vi "Open.vi"(8 "error in (no error)":errorcluster, 10 "address":string, 11 "Inst.Xeryon-Rotator in":refnum<class "Inst.Xeryon-Rotator.lvclass">) -> (0 "error out":errorcluster, 3 "Inst.Xeryon-Rotator out":refnum<class "Inst.Xeryon-Rotator.lvclass">)   [LabVIEW 2019, in "Inst.Xeryon-Rotator.lvclass"]
uses:
  Inst.Xeryon-Rotator.lvclass
  <userlib>/LevyLab/Instrument Framework/Instrument/Instrument.lvclass
  <userlib>/LevyLab/Instrument Framework/Instrument Types/Cryostat/Instrument.Cryostat.lvclass
  C:/Program Files (x86)/National Instruments/LabVIEW 2019/user.lib/LevyLab/Instrument Framework/Instrument Types/Cryostat/Instrument.Cryostat.lvclass
  C:/Program Files (x86)/National Instruments/LabVIEW 2019/user.lib/LevyLab/Instrument Framework/Instrument/Instrument.lvclass
  C:/Program Files (x86)/National Instruments/LabVIEW 2019/vi.lib/JKI/JKI SMO/SMO/SMO.lvclass
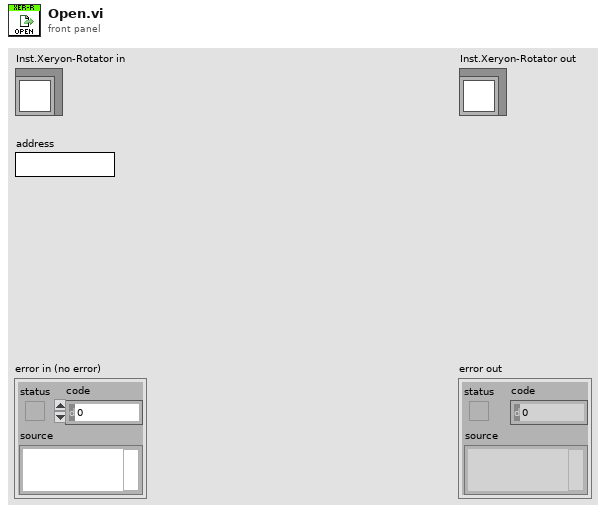
[diagram p1: front panel]
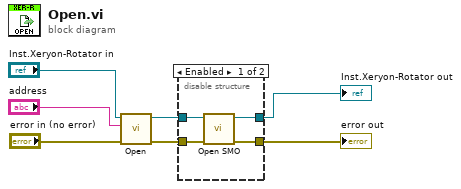
[diagram p0: block diagram]
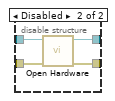
[diagram p2: hidden frame]
diagram:
  n1 = call-parent "Open.vi"("error in (no error)"="error in (no error)", "address"="address", "Instrument in"="Inst.Xeryon-Rotator in") -> ("error out"=w4:errorcluster, "Instrument out"=w3:refnum<class "Inst.Xeryon-Rotator.lvclass">)  [unwired: 7 in]
  n2 = disable-structure shown="Enabled" {
    disable-tunnel: w4 -> [w11 w14]
    disable-tunnel: w3 -> [w10 w15]
    disable-tunnel: [w9 w13] -> w2
    disable-tunnel: [w8 w12] -> w1
    frame Enabled {
      n3 = call <userlib>:"Open SMO.vi"("error in (no error)"=w11, "Instrument in"=w10) -> ("error out"=w8:errorcluster, "Instrument out"=w9:refnum<class "Inst.Xeryon-Rotator.lvclass">)  [unwired: 8 in]
    }
    frame Disabled {
      n4 = call-dynamic "Open Hardware.vi"("error in (no error)"=w14, "Inst.Xeryon-Rotator in"=w15) -> ("error out"=w12:errorcluster, "Inst.Xeryon-Rotator out"=w13:refnum<class "Inst.Xeryon-Rotator.lvclass">)  [unwired: 8 in]
    }
  }
  "error out" <- w1
  "Inst.Xeryon-Rotator out" <- w2
